vi "FullMermaidParse.vi"(8 "error in (no error)":errorcluster, 11 "ParseMermaid in":refnum<class "ParseMermaid.lvclass">) -> (0 "error out":errorcluster, 3 "ParseMermaid out":refnum<class "ParseMermaid.lvclass">)   [LabVIEW 2020, in "Mermaid.lvlib" / "ParseMermaid.lvclass"]
uses:
  ParseMermaid.lvclass
  ParseMermaid.lvclass/ParseMermaid.ctl
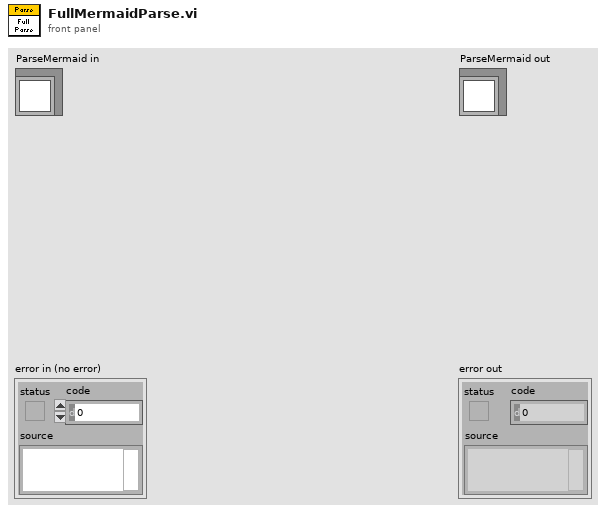
[diagram p1: front panel]
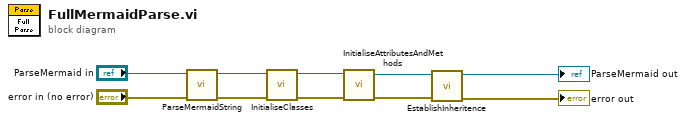
[diagram p0: block diagram]
diagram:
  n1 = call "ParseMermaidString.vi"("error in (no error)"="error in (no error)", "ParseMermaid in"="ParseMermaid in") -> ("error out"=w9:errorcluster, "ParseMermaid out"=w10:refnum<class "ParseMermaid.lvclass">)  [unwired: 8 in]
  n2 = call "InitialiseClasses.vi"("error in (no error)"=w9, "ParseMermaid in"=w10) -> ("error out"=w7:errorcluster, "ParseMermaid out"=w8:refnum<class "ParseMermaid.lvclass">)  [unwired: 8 in]
  n3 = call "InitialiseAttributesAndMethods.vi"("error in (no error)"=w7, "ParseMermaid in"=w8) -> ("error out"=w5:errorcluster, "ParseMermaid out"=w6:refnum<class "ParseMermaid.lvclass">)  [unwired: 8 in]
  n4 = call "EstablishInheritence.vi"("error in (no error)"=w5, "ParseMermaid in"=w6) -> ("error out"=→"error out":errorcluster, "ParseMermaid out"=→"ParseMermaid out":refnum<class "ParseMermaid.lvclass">)  [unwired: 8 in]
